vi "Destroy.vi"(0 "reference in":refnum<class "Reporter.lvclass">, 5 "error in (no error)":errorcluster) -> (14 "reference out":refnum<class "Reporter.lvclass">, 19 "error out":errorcluster)   [LabVIEW 2018, in "Reporter.lvclass"]
uses:
  Reporter.lvclass
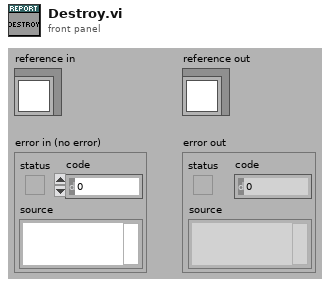
[diagram p1: front panel]
types:
  T1 = typedef "Reporter.lvclass/ObjectAttributes.ctl" = cluster{"Attribute1":dbl}
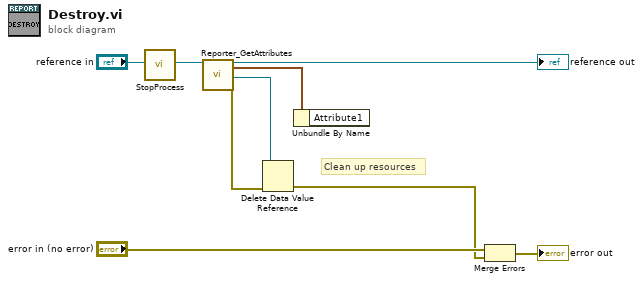
[diagram p0: block diagram]
diagram:
  # "Clean up resources"
  n1 = call "StopProcess.vi"("reference in"="reference in") -> ("reference out"=w1:refnum<class "Reporter.lvclass">)  [unwired: 17 in, 1 out]
  n2 = call "Reporter_GetAttributes.vi"("reference in"=w1) -> ("reference out"=→"reference out":refnum<class "Reporter.lvclass">, "Data"=w5:T1, "DataRef"=w6:refnum<data-value>, "error out"=w7:errorcluster)  [unwired: 15 in]
  n3 = Delete Data Value Reference(data value reference=w6, error in=w7) -> (error out=w3:errorcluster)  [unwired: 1 out]
  n4 = Unbundle By Name(w5) -> ()  [unwired: 1 out]
  n5 = Merge Errors("error in (no error)", w3) -> (→"error out":errorcluster)
